vi "catalog.get_dataset.path.vi"(8 "error in":errorcluster, 11 "Dataset UUID":string) -> (0 "error out":errorcluster, 2 "path":string)   [LabVIEW 2020, in "Nominal Client.lvclass"]
uses:
  Nominal Client.lvclass
  Nominal Client.lvclass/Nominal Client.ctl
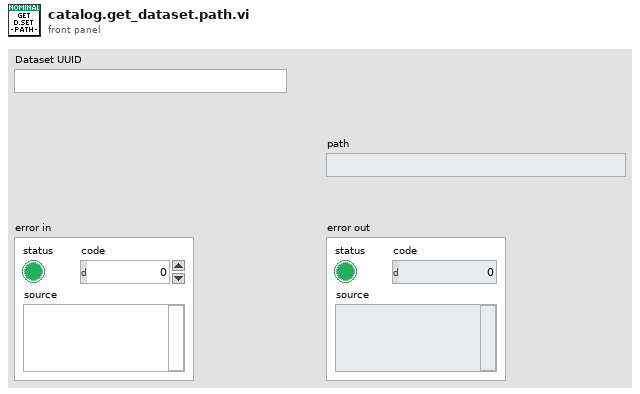
[diagram p1: front panel]
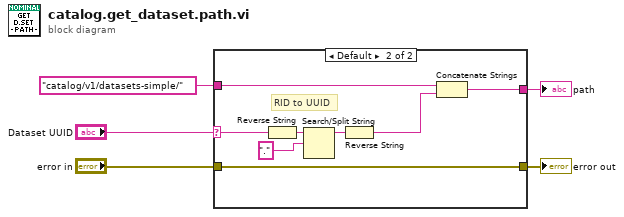
[diagram p0: block diagram]
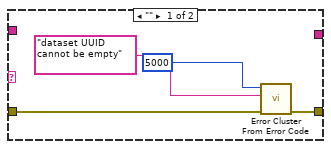
[diagram p2: hidden frame]
diagram:
  n1 = case shown="Default" "Dataset UUID" {
    selector: "Dataset UUID" -> [_ w11]
    tunnel: "catalog/v1/datasets-simple/" ("path") -> [_ w15]
    tunnel: [_ w17] -> w4
    tunnel: "error in" -> [w6 w16]
    tunnel: [w8 w16] -> w1
    frame "" {
      n2 = call <vilib>:"Error Cluster From Error Code.vi"("error in (no error)"=w6, "error message (\"\")"="dataset UUID cannot be empty" ("error message (\"\")"), "error code (0)"=5000) -> ("error out"=w8:errorcluster)  [unwired: 6 in]
    }
    frame Default {
      # "RID to UUID"
      n3 = Reverse String(1:w11) -> (0:w14:string)
      n4 = Search/Split String(string=w14, search string/char (-)=".") -> (substring before match=w12:string)  [unwired: 1 in, 2 out]
      n5 = Reverse String(1:w12) -> (0:w10:string)
      n6 = Concatenate Strings(w15, w10) -> (w17:string)
    }
  }
  "path" <- w4
  "error out" <- w1
